vi "VIName.vi"(7 "FullName":bool=TRUE, 11 "reference":refnum<vi>) -> (2 "filename without extension":string, 3 "VI Name":string)   [LabVIEW 2021]
doc: "Get the VI's Name, Fot error Handle or otherthings.\n20140302；\njiangsong@outlook.com"
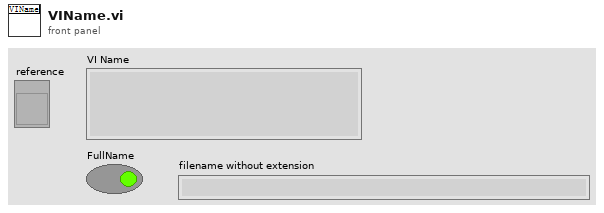
[diagram p1: front panel]
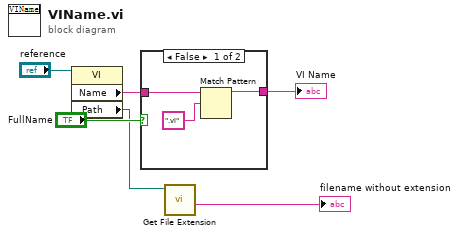
[diagram p0: block diagram]
diagram:
  n1 = property class="VI"(reference="reference") -> ("Name"=w5:string, "Path"=w2:path)  [unwired: 1 in, 2 out]
  n2 = case shown="False" "FullName" {
    tunnel: w5 -> [w8 w10]
    tunnel: [w7 w10] -> w4
    frame False {
      n3 = Match Pattern(string=w8, regular expression=".vi") -> (before substring=w7:string)  [unwired: 1 in, 3 out]
    }
    frame True {
    }
  }
  "VI Name" <- w4
  n4 = call <vilib>:"Get File Extension.vi"("file"=w2) -> ("filename without extension"=→"filename without extension":string)  [unwired: 6 in, 4 out]
